vi "gfitsio-get-num-keys.vi"(8 "error in (no error)":errorcluster, 11 "gfits refnum":T1) -> (0 "error out":errorcluster, 2 "number of keys":i32, 3 "dup gfits refnum":T1)   [LabVIEW 2015]
doc: "Return the number of existing keywords (not counting the END keyword)."
uses:
  gfitsio-refnum.ctl
  gfitsio.dll
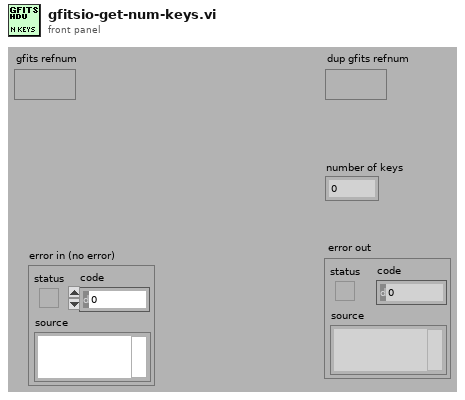
[diagram p1: front panel]
types:
  T1 = typedef "gfitsio-refnum.ctl" = refnum<k1>
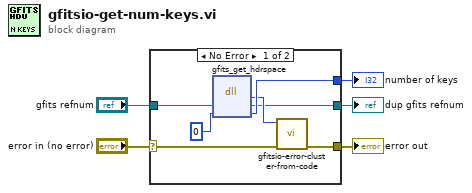
[diagram p0: block diagram]
diagram:
  n1 = case shown="No Error" "error in (no error)" {
    selector: "error in (no error)" -> [w10 w14]
    tunnel: [w9 w14] -> w5
    tunnel: "gfits refnum" -> [w7 w13]
    tunnel: [w8 w13] -> w3
    tunnel: [w12 _] -> w1
    frame No Error {
      n2 = dll-call lib="C:/ALPHA GSCS/GSCS/Systems/SIcamera_Control/Quick_Look/gfitsio/gfitsio.dll" fn="gfits_get_hdrspace"("gfits refnum"=w7, "nexist"=0) -> (w11:i32, "gfits refnum"=w8:T1, "nexist"=w12:i32)  [unwired: 3 in, 2 out]
      n3 = call "gfitsio-error-cluster-from-code.vi"("error in (no error)"=w10, "error code"=w11) -> ("error out"=w9:errorcluster)  [unwired: 9 in]
    }
    frame Error {
    }
  }
  "error out" <- w5
  "dup gfits refnum" <- w3
  "number of keys" <- w1
